vi "HP E3633A set volts.vi"(8 "Voltage":dbl, 11 "VISA resource name":refnum<visa-resource-name>) -> ()   [LabVIEW 2015]
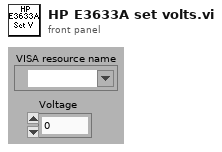
[diagram p1: front panel]
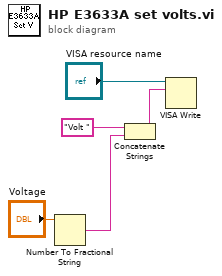
[diagram p0: block diagram]
diagram:
  n1 = Number To Fractional String(number="Voltage") -> (F-format string=w2:string)  [unwired: 3 out]
  n2 = Concatenate Strings("Volt " ("write buffer"), w2) -> (w3:string)
  n3 = VISA Write(VISA resource name="VISA resource name", write buffer=w3) -> ()  [unwired: 1 in, 3 out]
